vi "Begin.vi"(8 "error in":errorcluster) -> (0 "error out":errorcluster)   [LabVIEW 2015]
doc: "Called before other user functions, this VI is expected to open initial I/O refnums, load in file data, and do all program initialization. Notice that the <B>error out</B> terminal is simply used for data flow. Wiring it to other structures or subVIs ensures that this VI runs first."
uses:
  <vilib>/Rock Robotics/SystemInterfaces/DIO/FPGA_DIOPWMChannel.ctl
  <vilib>/Rock Robotics/WPI/SafetyOutput/WPI_SafetyOutputConfigMenu.ctl
  <vilib>/Rock Robotics/WPI/DriverStation/WPI_DriverStationRobotMode2.ctl
  <vilib>/Rock Robotics/WPI/Joystick/WPI_JoystickDeviceEnum.ctl
  <vilib>/Rock Robotics/WPI/Solenoid/WPI_SolenoidChannel.ctl
  <vilib>/Rock Robotics/WPI/AnalogOutput/WPI_AnalogOutputChannel.ctl
  <vilib>/Rock Robotics/WPI/RobotDrive/WPI_RobotDriveOpen2MotorWithTalon.vi
  Robot Global Data.vi
  <vilib>/Rock Robotics/Network Tables/SD Write String Array.vi
  <vilib>/Rock Robotics/WPI/Solenoid/WPI_SolenoidOpenDouble.vi
  <vilib>/Rock Robotics/WPI/Solenoid/WPI_SolenoidOpenSingle.vi
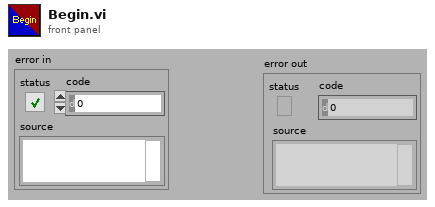
[diagram p1: front panel]
types:
  T1 = typedef "WPI_SolenoidChannel.ctl" = enum8{"Solenoid 0", "Solenoid 1", "Solenoid 2", "Solenoid 3", "Solenoid 4", "Solenoid 5", "Solenoid 6", "Solenoid 7", "Invalid"}
  T2 = typedef "WPI_AnalogOutputChannel.ctl" = enum8{"AO MXP 0", "AO MXP 1", "Invalid"}
  T3 = typedef "FPGA_DIOPWMChannel.ctl" = enum8{"PWM 0", "PWM 1", "PWM 2", "PWM 3", "PWM 4", "PWM 5", "PWM 6", "PWM 7", "PWM 8", "PWM 9", "PWM MXP 0", "PWM MXP 1", "PWM MXP 2", "PWM MXP 3", "PWM MXP 4", "PWM MXP 5", "PWM MXP 6", "PWM MXP 7", "PWM MXP 8", "PWM MXP 9", "Invalid"}
  T4 = typedef "WPI_JoystickDeviceEnum.ctl" = enum16{"USB 0", "USB 1", "USB 2", "USB 3", "USB 4", "USB 5"}
  T5 = typedef "WPI_DriverStationRobotMode2.ctl" = enum16{"Autonomous Disabled", "Autonomous Enabled", "Teleop Disabled", "Teleop Enabled", "Disconnected", "Finish", "Test Disabled", "Test Enabled", "Emergency Stopped"}
  T6 = typedef "WPI_SafetyOutputConfigMenu.ctl" = enum16{"Enable", "Disable"}
  T7 = typedef "WPI_JoystickDevRef.ctl" = cluster{"Device":T4}
  T8 = typedef "WPI_SolenoidDevRef.ctl" = cluster{"DevStatus":errorcluster, "Pneumatics Control Module":u8, "Forward Solenoid Channel":T1, "Reverse Solenoid Channel":T1}
  T9 = typedef "WPI_ServoDeviceRef.ctl" = cluster{"DeviceStatus":errorcluster, "PWM Channel":T3, "DeadBand":T10}
  T10 = typedef "WPI_PWMDeadband.ctl" = cluster{"Name":string, "maxPositivePwm":i32, "minPositivePwm":i32, "centerPwm":i32, "maxNegativePwm":i32, "minNegativePwm":i32, "angularRange":u16}
  T11 = typedef "WPI_AOChannelDevRef.ctl" = cluster{"DevStatus":errorcluster, "AO Channel":T2}
  T12 = typedef "WPI_RobotDriveDevRef.ctl" = cluster{"DevStatus":errorcluster, "Motors[]":T13[], "Square Inputs":bool, "Max Output":dbl}
  T13 = typedef "WPI_MotorControlDeviceRef.ctl" = cluster{"DeviceStatus":errorcluster, "Type":T14, "PWM":cluster{"PWM Channel":T3, "DeadBand":T10}, "CAN":cluster{"Device Number":u8, "Control Mode":T15, "Semaphore":T16, "Max Vout":dbl, "TalonSRX Control Mode":T17}, "Invert":bool}
  T14 = typedef "WPI_MotorControlType.ctl" = enum16{"PWM", "CAN", "CANTalonSRX"}
  T15 = typedef "WPI_CANJaguar_ControlMode.ctl" = enum8{"Percent VBus", "Current", "Speed", "Position", "Voltage"}
  T16 = typedef "Semaphore RefNum" = refnum<k1>
  T17 = typedef "WPI_CANTalonSRX_APIControlMode.ctl" = enum8{"Percent VBus", "Speed", "Position", "Slave", "Unchanged / Invalid", "Voltage Compensation", "Current", "Motion Profile"}
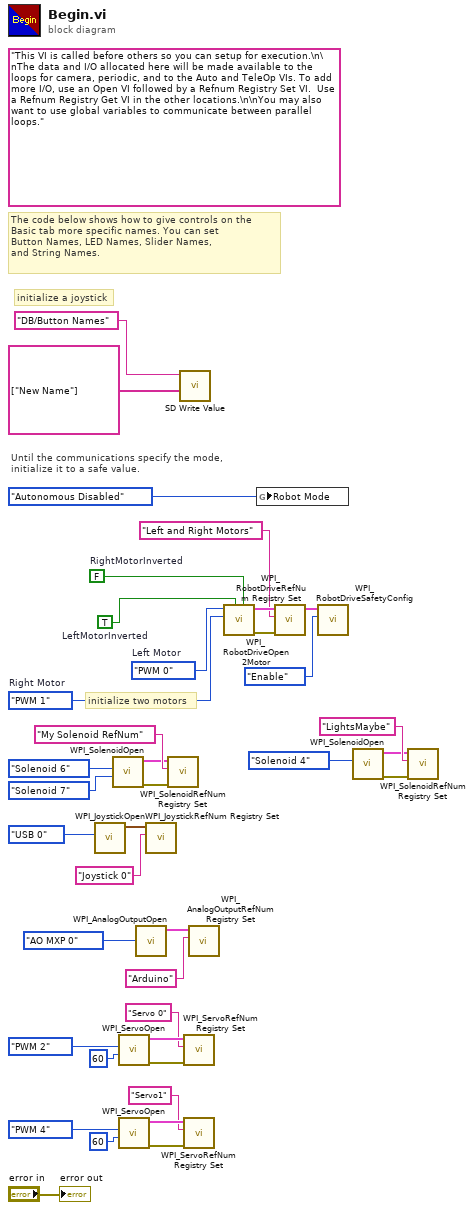
[diagram p0: block diagram]
diagram:
  (unwired) "This VI is called before others so you can setup for execution.\n\nThe data and I/O allocated here will be made available to the loops for camera, periodic, and to the Auto and TeleOp VIs. To add more I/O, use an Open VI followed by a Refnum Registry Set VI.  Use a Refnum Registry Get VI in the other locations.\n\nYou may also want to use global variables to communicate between parallel loops."
  w32 = FPGA_DIOPWMChannel."PWM 1"  # Right Motor
  w33 = FPGA_DIOPWMChannel."PWM 0"  # Left Motor
  w37 = TRUE  # LeftMotorInverted
  w38 = FALSE  # RightMotorInverted
  # "The code below shows how to give controls on the\nBasic tab more specific names. You can set\nButton Names, LED Names, Slider Names,\nand String Names."
  # "initialize a joystick"
  # "Until the communications specify the mode,\ninitialize it to a safe value."
  # "initialize two motors"
  n1 = call <vilib>:"WPI_JoystickOpen.vi"("JoystickDevice"=WPI_JoystickDeviceEnum."USB 0") -> ("JoystickDevRef"=w27:T7)  [unwired: 10 in]
  n2 = call-poly <vilib>:"WPI_SolenoidOpen.vi"("Reverse Solenoid Channel"=WPI_SolenoidChannel."Solenoid 7", "Forward Solenoid Channel"=WPI_SolenoidChannel."Solenoid 6") -> ("error out"=w8:errorcluster, "SolenoidDevRef"=w9:T8)  [unwired: 8 in]
  n3 = call <vilib>:"WPI_ServoOpen.vi"("Angular Range"=u16 60, "PWM Channel"=FPGA_DIOPWMChannel."PWM 2") -> ("error out"=w16:errorcluster, "ServoDeviceRef"=w17:T9)  [unwired: 8 in]
  n4 = call <vilib>:"WPI_ServoOpen.vi"("Angular Range"=u16 60, "PWM Channel"=FPGA_DIOPWMChannel."PWM 4") -> ("error out"=w11:errorcluster, "ServoDeviceRef"=w12:T9)  [unwired: 8 in]
  n5 = call <vilib>:"WPI_AnalogOutputOpen.vi"("AO Channel"=WPI_AnalogOutputChannel."AO MXP 0") -> ("AODeviceRef"=w5:T11)  [unwired: 9 in, 1 out]
  n6 = call <vilib>:"WPI_JoystickRefNum Registry Set.vi"("refnum name"="Joystick 0", "JoystickDevRef"=w27) -> ()  [unwired: 8 in, 2 out]
  n7 = call <vilib>:"WPI_SolenoidRefNum Registry Set.vi"("error in (no error)"=w8, "refnum name"="My Solenoid RefNum", "SolenoidDevRef"=w9) -> ()  [unwired: 7 in, 2 out]
  n8 = call-poly <vilib>:"SD Write Value.vi"("String Array"=string[] ["New Name"], "Name"="DB/Button Names") -> ()  [unwired: 8 in, 2 out]
  n9 = call <vilib>:"WPI_ServoRefNum Registry Set.vi"("error in (no error)"=w16, "refnum name"="Servo 0", "ServoDeviceRef"=w17) -> ()  [unwired: 7 in, 2 out]
  n10 = call <vilib>:"WPI_ServoRefNum Registry Set.vi"("error in (no error)"=w11, "refnum name"="Servo1", "ServoDeviceRef"=w12) -> ()  [unwired: 7 in, 2 out]
  n11 = call <vilib>:"WPI_AnalogOutputRefNum Registry Set.vi"("refnum name"="Arduino", "AODeviceRef"=w5) -> ()  [unwired: 8 in, 2 out]
  n12 = call-poly <vilib>:"WPI_RobotDriveOpen2Motor.vi"("Right Motor Inverted"=w38, "Left Motor Inverted"=w37, "Right Motor"=w32, "Left Motor"=w33) -> ("error out"=w34:errorcluster, "RobotDriveDevRef"=w36:T12)  [unwired: 1 in, 5 out]
  n13 = global write "Robot Global Data.vi" "Robot Mode"(WPI_DriverStationRobotMode2."Autonomous Disabled" ("Robot Mode")) -> ()
  n14 = call <vilib>:"WPI_RobotDriveRefNum Registry Set.vi"("error in (no error)"=w34, "refnum name"="Left and Right Motors", "RobotDriveDevRef"=w36) -> ("RobotDriveDevRef"=w31:T12)  [unwired: 1 in, 7 out]
  n15 = call <vilib>:"WPI_RobotDriveSafetyConfig.vi"("mode"=WPI_SafetyOutputConfigMenu."Enable", "RobotDriveDevRef"=w31) -> ()  [unwired: 8 in, 2 out]
  n16 = call-poly <vilib>:"WPI_SolenoidOpen.vi"("Solenoid Channel"=WPI_SolenoidChannel."Solenoid 4" ("Forward Solenoid Channel")) -> ("error out"=w1:errorcluster, "SolenoidDevRef"=w2:T8)  [unwired: 9 in]
  n17 = call <vilib>:"WPI_SolenoidRefNum Registry Set.vi"("error in (no error)"=w1, "refnum name"="LightsMaybe", "SolenoidDevRef"=w2) -> ()  [unwired: 7 in, 2 out]
  "error out" <- "error in"
